vi "Controller 1.vi"(1 "Joystick Multiplier":dbl=1.0) -> (0 "Values":T1)   [LabVIEW 2013]
uses:
  <vilib>/Rock Robotics/WPI/Joystick/WPI_JoystickGetSetRefNum.vi
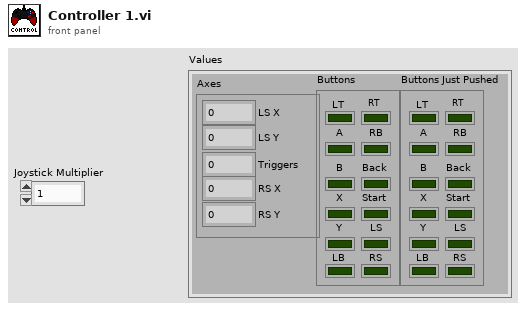
[diagram p1: front panel]
types:
  T1 = cluster{"Axes":cluster{"LS X":dbl, "LS Y":dbl, "Triggers":dbl, "RS X":dbl, "RS Y":dbl}, "Buttons":cluster{"LT":bool, "RT":bool, "A":bool, "B":bool, "X":bool, "Y":bool, "LB":bool, "RB":bool, "Back":bool, "Start":bool, "LS":bool, "RS":bool}, "Buttons Just Pushed":cluster{"LT":bool, "RT":bool, "A":bool, "B":bool, "X":bool, "Y":bool, "LB":bool, "RB":bool, "Back":bool, "Start":bool, "LS":bool, "RS":bool}}
  T2 = typedef "WPI_JoystickDevRef.ctl" = cluster{"Device":T3}
  T3 = typedef "WPI_JoystickDeviceEnum.ctl" = enum16{"USB 1", "USB 2", "USB 3", "USB 4", "Kinect 1", "Kinect 2"}
  T4 = typedef "WPI_JoystickButtonState.ctl" = cluster{"Button 1":bool, "Button 2":bool, "Button 3":bool, "Button 4":bool, "Button 5":bool, "Button 6":bool, "Button 7":bool, "Button 8":bool, "Button 9":bool, "Button 10":bool, "Button 11":bool, "Button 12":bool}
  T5 = cluster{"axis 1 (x)":dbl, "axis 2 (y)":dbl, "axis 3 (throttle)":dbl, "axis 4":dbl, "axis 5":dbl, "axis 6":dbl}
  T6 = cluster{"axis 1 (x)":dbl, "axis 2 (y)":dbl, "axis 3 (throttle)":dbl, "axis 4":dbl, "axis 5":dbl}
  T7 = cluster{bool, bool, "Button 1":bool, "Button 2":bool, "Button 3":bool, "Button 4":bool, "Button 5":bool, "Button 6":bool, "Button 7":bool, "Button 8":bool, "Button 9":bool, "Button 10":bool}
  T8 = cluster{"[0]":dbl, "[1]":dbl, "[2]":dbl, "[3]":dbl, "[4]":dbl}
  T9 = cluster{cluster{"[0]":dbl, "[1]":dbl, "[2]":dbl, "[3]":dbl, "[4]":dbl}, cluster{bool, bool, "Button 1":bool, "Button 2":bool, "Button 3":bool, "Button 4":bool, "Button 5":bool, "Button 6":bool, "Button 7":bool, "Button 8":bool, "Button 9":bool, "Button 10":bool}, cluster{bool, bool, "Button 1":bool, "Button 2":bool, "Button 3":bool, "Button 4":bool, "Button 5":bool, "Button 6":bool, "Button 7":bool, "Button 8":bool, "Button 9":bool, "Button 10":bool}}
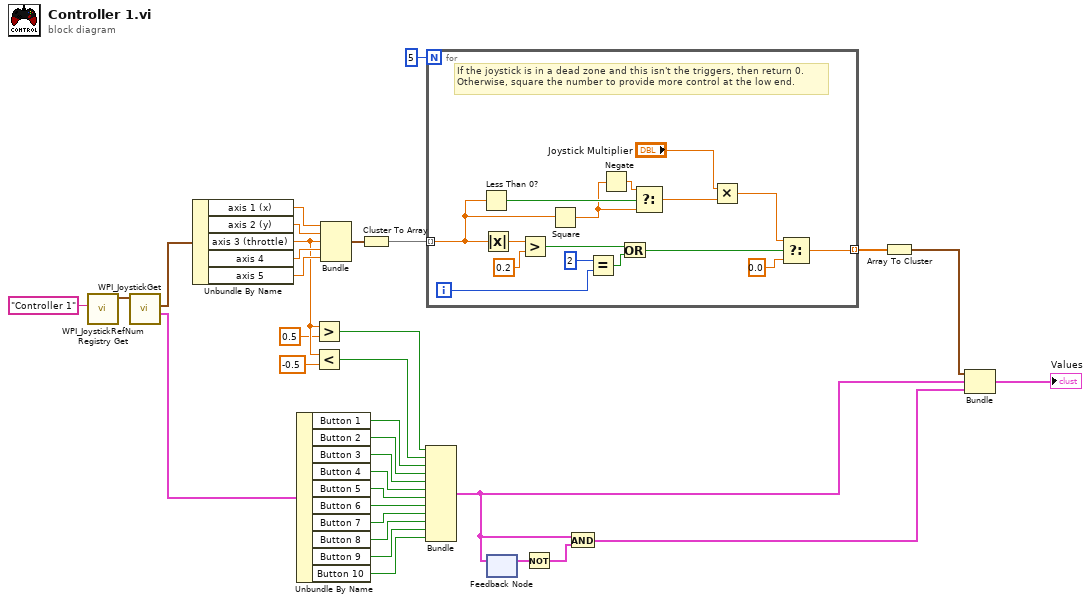
[diagram p0: block diagram]
diagram:
  n1 = call <vilib>:"WPI_JoystickRefNum Registry Get.vi"("refnum name"="Controller 1") -> ("JoystickDevRef"=w33:T2)  [unwired: 9 in, 1 out]
  n2 = call <vilib>:"WPI_JoystickGet.vi"("JoystickDevRef"=w33) -> ("Buttons"=w6:T4, "Axes"=w22:T5)  [unwired: 4 in, 1 out]
  n3 = Unbundle By Name(w22) -> ("axis 1 (x)"=w21:dbl, "axis 2 (y)"=w20:dbl, "axis 3 (throttle)"=w11:dbl, "axis 4"=w19:dbl, "axis 5"=w18:dbl)
  n4 = Unbundle By Name(w6) -> ("Button 1"=w32:bool, "Button 2"=w31:bool, "Button 3"=w30:bool, "Button 4"=w29:bool, "Button 5"=w28:bool, "Button 6"=w27:bool, "Button 7"=w26:bool, "Button 8"=w25:bool, "Button 9"=w24:bool, "Button 10"=w23:bool)
  n5 = Greater?(x=w11, y=0.5) -> (0:w12:bool)
  n6 = Less?(x=w11, y=-0.5) -> (x < y?=w8:bool)
  n7 = Bundle("axis 1 (x)"=w21, "axis 2 (y)"=w20, "axis 3 (throttle)"=w11, "axis 4"=w19, "axis 5"=w18) -> (w16:T6)  [unwired: 1 in]
  n8 = Cluster To Array(cluster=w16) -> (array=w15:dbl[])
  n9 = Bundle(w12, w8, "Button 1"=w32, "Button 2"=w31, "Button 3"=w30, "Button 4"=w29, "Button 5"=w28, "Button 6"=w27, "Button 7"=w26, "Button 8"=w25, "Button 9"=w24, "Button 10"=w23) -> (w3:T7)  [unwired: 1 in]
  n10 = for {
    N: 5 -> [_]
    tunnel: w15 -> [w44] mode=indexing
    tunnel: [w47] -> w14 mode=indexing
    i -> [w38]
    # "If the joystick is in a dead zone and this isn't the triggers, then return 0.\nOtherwise, square the number to provide more control at the low end."
    n11 = Less Than 0?(x=w44) -> (x < 0?=w45:bool)
    n12 = Absolute Value(x=w44) -> (abs(x)=w46:dbl)
    n13 = Greater?(x=w46, y=0.2) -> (0:w41:bool)
    n14 = Square(x=w44) -> (x^2=w43:dbl)
    n15 = Equal?(x=2, y=w38) -> (x = y?=w39:bool)
    n16 = Negate(x=w43) -> (-x=w42:dbl)
    n17 = Or(x=w41, y=w39) -> (x .or. y?=w40:bool)
    n18 = Select(t=w42, s=w45, f=w43) -> (s? t:f=w35:dbl)
    n19 = Multiply(x="Joystick Multiplier", y=w35) -> (x*y=w36:dbl)
    n20 = Select(t=w36, s=w40, f=0.0) -> (s? t:f=w47:dbl)
  }
  n21 = feedback #1() -> (w7:T7)  [unwired: 1 in]
  n22 = feedback-in #1(w3) -> ()
  n23 = Not(x=w7) -> (.not. x?=w5:T7)
  n24 = And(x=w3, y=w5) -> (x .and. y?=w2:T7)
  n25 = Array To Cluster(array=w14) -> (cluster=w4:T8)
  n26 = Bundle(w4, w3, w2) -> (→"Values":T9)  [unwired: 1 in]
